vi "Choo Choo Shoot.vi"(8 "error in":errorcluster) -> (0 "error out":errorcluster)   [LabVIEW 2014]
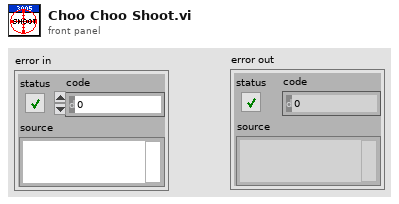
[diagram p1: front panel]
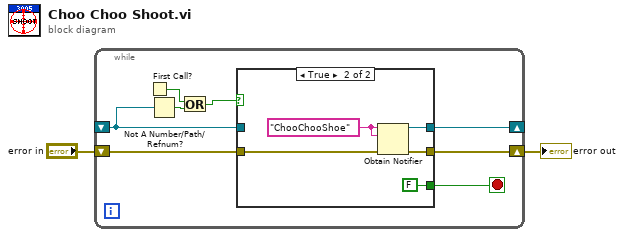
[diagram p0: block diagram]
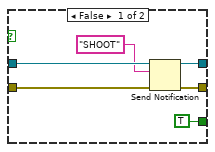
[diagram p2: hidden frame]
diagram:
  n1 = while {
    shift-right: [w10] -> _
    shift-left: _ -> [w6]
    shift-right: [w9] -> w2
    shift-left: "error in" -> [w8]
    stop <- w7 stop-if-true
    n2 = First Call?() -> (First Call?: T/F=w3:bool)
    n3 = Not A Number/Path/Refnum?(number/path/refnum=w6) -> (NaN/Path/Refnum?=w4:bool)
    n4 = Or(x=w3, y=w4) -> (x .or. y?=w5:bool)
    n5 = case shown="True" w5 {
      tunnel: [w15 w20] -> w10
      tunnel: w6 -> [w16 _]
      tunnel: [w13 w18] -> w9
      tunnel: w8 -> [w12 w19]
      tunnel: [TRUE FALSE] -> w7
      frame False {
        n6 = Send Notification(notification="SHOOT" ("name (unnamed)"), notifier=w16, error in (no error)=w12) -> (notifier out=w15:refnum<notifier>, error out=w13:errorcluster)
      }
      frame True {
        w21 = "ChooChooShoe" ("name (unnamed)")
        n7 = Obtain Notifier(name (unnamed)=w21, notification data type=w21, error in (no error)=w19) -> (notifier out=w20:refnum<notifier>, error out=w18:errorcluster)  [unwired: 1 in, 1 out]
      }
    }
  }
  "error out" <- w2
